vi "Call Subpanel VI.vi"(8 "error in (no error)":errorcluster, 10 "VI Refnum":refnum<vi>, 11 "Motor Configuration in":refnum<class "Motor Configuration.lvclass">) -> (0 "error out":errorcluster, 3 "Motor Configuration out":refnum<class "Motor Configuration.lvclass">)   [LabVIEW 2016, in "Hardware.lvlib" / "Motor.lvlib" / "Motor Configuration.lvclass"]
uses:
  <userlib>/Common Components/Hardware/Motor/Motor Config/Motor Configuration.lvclass
  <userlib>/Configuration Dialog Actor/Configuration.lvclass
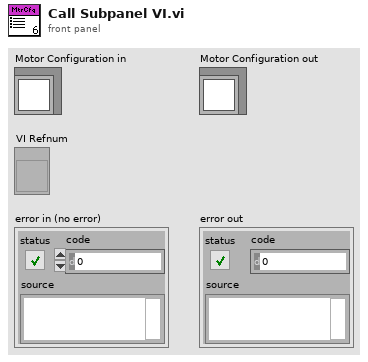
[diagram p1: front panel]
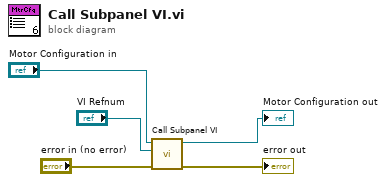
[diagram p0: block diagram]
diagram:
  n1 = call-parent "Call Subpanel VI.vi"("error in (no error)"="error in (no error)", "VI Refnum"="VI Refnum", "Configuration in"="Motor Configuration in") -> ("error out"=→"error out":errorcluster, "Configuration out"=→"Motor Configuration out":refnum<class "Motor Configuration.lvclass">)  [unwired: 7 in]
